vi "GenerateConfig.vi"() -> (3 "JSON string":string)   [LabVIEW 2017, in "MQTT.lvlib"]
uses:
  MQTT.lvlib
  OOP/config.ctl
  OOP/MQTTclient.lvclass
panel:
  in  "Load":bool=TRUE
  in  "SAVE":bool=TRUE
  in  "OK":bool=TRUE
  in  "Config":T1={"Broker"={"IP"="192.168.", "port"=1883, "connTimeout"=3000, "writeTimeout"=3000, "readTimeout"=3000, "subTimeout"=3000}, "Connect Flags"={"reserved"=FALSE, "clean session"=FALSE, "will flag"=FALSE, "willQOS"="At least once", "will retain"=FALSE, "password"=FALSE, "user name"=FALSE}, "Keep Alive"=0, "Client Info"={"ClientId"="", "Will Topic"="", "Will Message"="", "User Name"="", "Password"=""}}
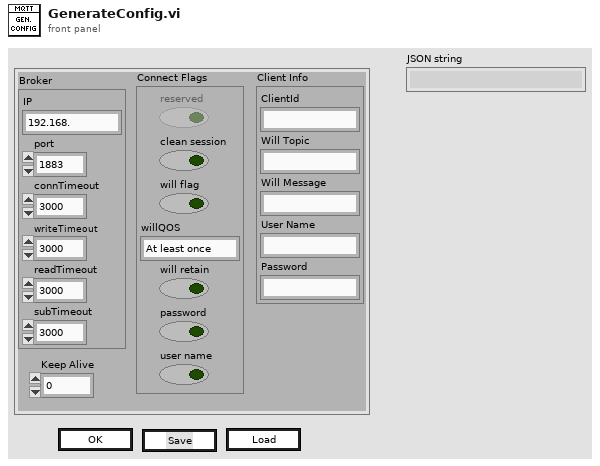
[diagram p1: front panel]
types:
  T1 = typedef "MQTTclient.lvclass/config.ctl" = cluster{"Broker":cluster{"IP":string, "port":u16, "connTimeout":i32, "writeTimeout":i32, "readTimeout":i32, "subTimeout":i32}, "Connect Flags":cluster{"reserved":bool, "clean session":bool, "will flag":bool, "willQOS":string, "will retain":bool, "password":bool, "user name":bool}, "Keep Alive":u16, "Client Info":cluster{"ClientId":string, "Will Topic":string, "Will Message":string, "User Name":string, "Password":string}}
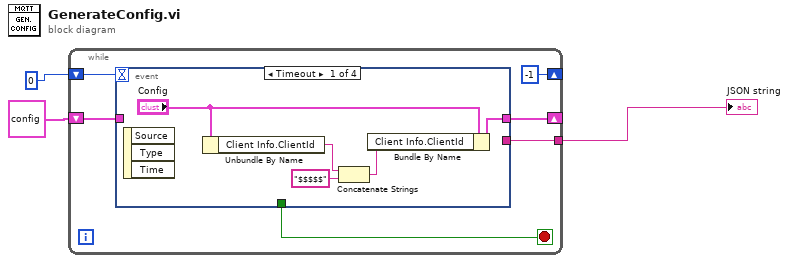
[diagram p0: block diagram]
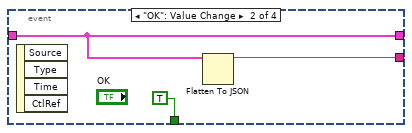
[diagram p2: hidden frame]
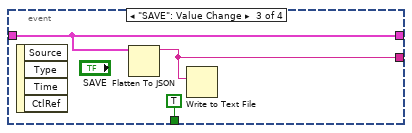
[diagram p3: hidden frame]
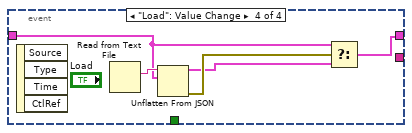
[diagram p4: hidden frame]
diagram:
  n1 = while {
    shift-right: [w9] -> _
    shift-left: T1 {"Broker"={"IP"="", "port"=1883, "connTimeout"=3000, "writeTimeout"=3000, "readTimeout"=3000, "subTimeout"=3000}, "Connect Flags"={"reserved"=FALSE, "clean session"=FALSE, "will flag"=FALSE, "willQOS"="At least once", "will retain"=FALSE, "password"=FALSE, "user name"=FALSE}, "Keep Alive"=0, "Client Info"={"ClientId"="", "Will Topic"="", "Will Message"="", "User Name"="", "Password"=""}} ("Config") -> [w8]
    tunnel: [w6] -> w3
    shift-right: [-1] -> _
    shift-left: 0 -> [w5]
    stop <- w7 stop-if-true
    n2 = event shown="[0] Timeout" {
      selector: _ -> [_ _ _ _]
      dyn-events: _ -> [_ _ _ _]
      timeout: w5 -> [_ _ _ _]
      tunnel: [w13 w16 w20 w21] -> w9
      tunnel: w8 -> [_ w16 w20 w23]
      tunnel: [_ TRUE TRUE _] -> w7
      tunnel: [_ w15 w19 _] -> w6
      event Timeout {
        n3 = event-data() -> ()  [unwired: 1 in, 3 out]
        n4 = Unbundle By Name("Config") -> ("Client Info.ClientId"=w12:string)
        n5 = Concatenate Strings(w12, "$$$$$" ("string")) -> (w11:string)
        n6 = Bundle By Name(cluster="Config", "Client Info.ClientId"=w11) -> (w13:T1)
      }
      event "OK": Value Change {
        n7 = event-data() -> ()  [unwired: 1 in, 4 out]
        n8 = Flatten To JSON(anything=w16) -> (JSON string=w15:string)  [unwired: 2 in, 1 out]
      }
      event "SAVE": Value Change {
        n9 = event-data() -> ()  [unwired: 1 in, 4 out]
        n10 = Flatten To JSON(anything=w20) -> (JSON string=w19:string)  [unwired: 2 in, 1 out]
        n11 = Write to Text File(text=w19) -> ()  [unwired: 3 in, 3 out]
      }
      event "Load": Value Change {
        n12 = event-data() -> ()  [unwired: 1 in, 4 out]
        n13 = Read from Text File() -> (text=w25:string)  [unwired: 4 in, 3 out]
        n14 = Unflatten From JSON(JSON string=w25, type and defaults=w23) -> (value=w22:T1, error out=w24:errorcluster)  [unwired: 5 in]
        n15 = Select(t=w23, s=w24, f=w22) -> (s? t:f=w21:T1)
      }
    }
  }
  "JSON string" <- w3
